vi "Set Temperature.vi"(6 "Channel":i32, 8 "error in (no error)":errorcluster, 9 "Rate (K/min)":dbl, 10 "Temperature (K)":dbl, 11 "instrument.PPMS in":refnum<class "instrument.PPMS1.lvclass">) -> (0 "error out":errorcluster, 3 "instrument.PPMS out":refnum<class "instrument.PPMS1.lvclass">)   [LabVIEW 2019, in "instrument.PPMS1.lvclass"]
uses:
  instrument.PPMS1.lvclass
  Typedefs/PPMS1.Commands-enum.ctl
  <userlib>/LevyLab/Levylab Instruments/Instrument Types/Cryostat/Typedefs/Set Temperature--cluster.ctl
  39bf8733-267b-4609-bdd0-242e71fc71c5.vi
  39bf8733-267b-4609-bdd0-242e71fc71c5.vi/b51f7172-eccd-4dbe-95c5-5f0eea371546.vi
  <userlib>/LevyLab/Levylab Instruments/SMOs/RemoteControl/API/Remote Client.vi
  <userlib>/LevyLab/Levylab Instruments/Instrument Types/Cryostat/Instrument.Cryostat.lvclass
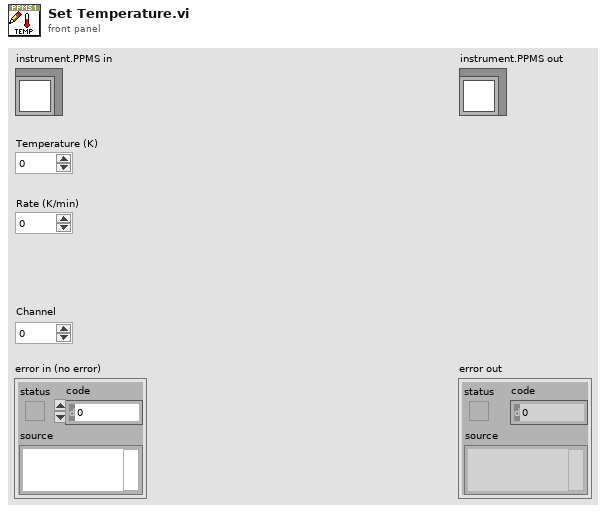
[diagram p1: front panel]
types:
  T1 = typedef "Instrument.Cryostat.lvclass/Set Temperature--cluster.ctl" = cluster{"Temperature (K)":dbl, "Rate (K/min)":dbl, "Channel":i32}
  T2 = typedef "instrument.PPMS1.lvclass/PPMS1.Commands-enum.ctl" = enum16{"Get Magnet Field", "Get Helium Level", "Get Temperature", "Set Magnet Field", "Set Temperature", "getAll"}
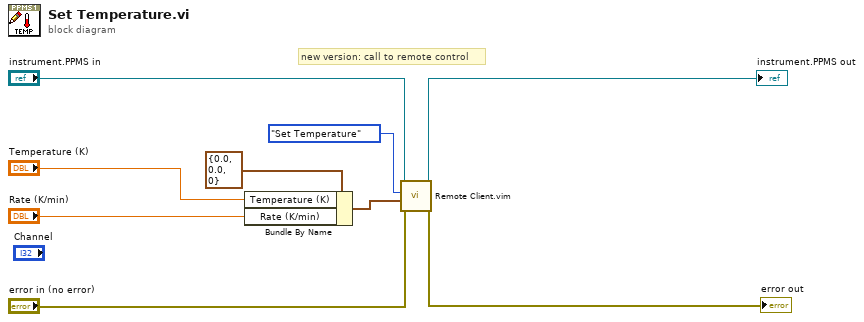
[diagram p0: block diagram]
diagram:
  # "new version: call to remote control"
  n1 = Bundle By Name(cluster=T1 {"Temperature (K)"=0.0, "Rate (K/min)"=0.0, "Channel"=0} ("Set Temperature"), "Temperature (K)"="Temperature (K)", "Rate (K/min)"="Rate (K/min)") -> (w3:T1)
  n2 = call "Remote Client.vim"("error in (no error)"="error in (no error)", "Data"=w3, "Command"=PPMS1.Commands-enum."Set Temperature", "Instrument in"="instrument.PPMS in") -> ("error out"=→"error out":errorcluster, "Instrument out"=→"instrument.PPMS out":refnum<class "instrument.PPMS1.lvclass">)  [unwired: 4 in, 2 out]
